vi "sub2.vi"(9 "Part References.Parse State Queue":refnum<vi>, 10 "regular expression":string, 11 "Array":T1(array[cluster])) -> (3 "Tunnel out":refnum<vi>)   [LabVIEW 2017, in "CSM-Helper.lvclass"]
doc: "### sub2.vi\n\n-- <b>Controls</b> --\n- <b>Part References.Parse State Queue</b>:\n- <b>regular expression</b>:\n- <b>Array</b>:\n\n-- <b>Indicators</b> --\n- <b>Tunnel out</b>:"
uses:
  CSM-Helper.lvclass
panel:
  # "Connector Pane"
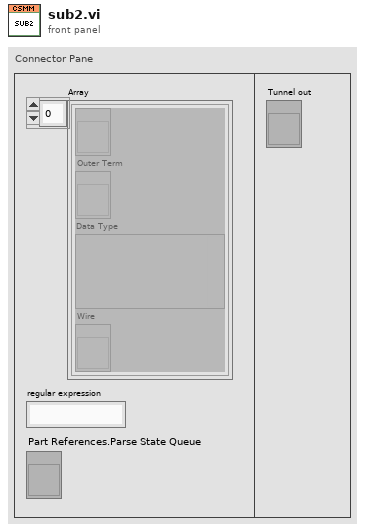
[diagram p1: front panel]
types:
  T1 = cluster{refnum<vi>, "Outer Term":refnum<vi>, "Data Type":variant, "Wire":refnum<vi>}[]
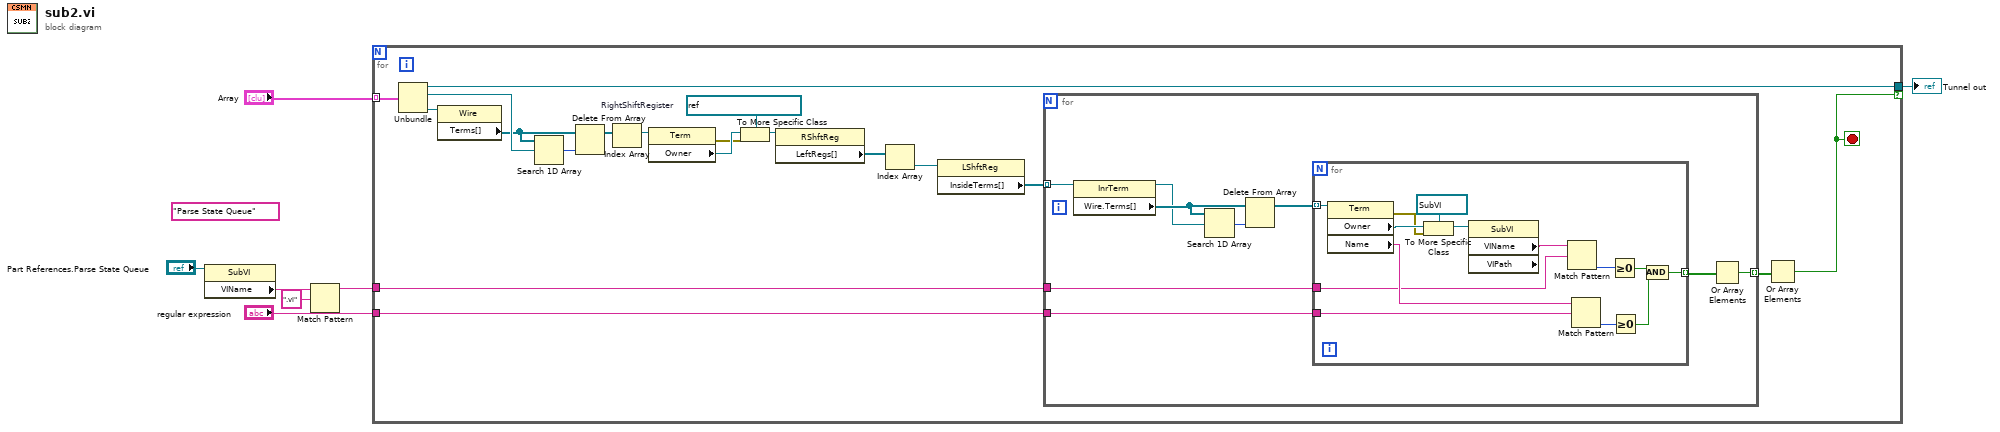
[diagram p0: block diagram]
diagram:
  (unwired) "Parse State Queue" ("regular expression")
  n1 = property class="SubVI"(reference="Part References.Parse State Queue") -> ("VIName"=w3:string)  [unwired: 1 in, 2 out]
  n2 = Match Pattern(string=w3, regular expression=".vi") -> (before substring=w2:string)  [unwired: 1 in, 3 out]
  n3 = for {
    tunnel: "Array" -> [w26] mode=indexing
    tunnel: [w25] -> w7 if=w16
    tunnel: "regular expression" -> [w15]
    tunnel: w2 -> [w8]
    stop <- w16 stop-if-true
    w22 = refnum<vi> refnum  # RightShiftRegister
    n4 = Unbundle(w26) -> (w25:refnum<vi>, "Outer Term"=w12:refnum<vi>, "Wire"=w24:refnum<vi>)  [unwired: 1 out]
    n5 = property class="Wire"(reference=w24) -> ("Terms[]"=w10:refnum<vi>[])  [unwired: 1 in, 2 out]
    n6 = Search 1D Array(1D array=w10, element=w12) -> (index of element=w11:i32)  [unwired: 1 in]
    n7 = Delete From Array(array=w10, index=w11) -> (array with subset deleted=w9:refnum<vi>[])  [unwired: 1 in, 1 out]
    n8 = Index Array(array=w9) -> (element=w23:refnum<vi>)  [unwired: 1 in]
    n9 = property class="Term"(reference=w23) -> (error out=w13:errorcluster, "Owner"=w14:refnum<vi>)  [unwired: 1 in, 1 out]
    n10 = To More Specific Class(target class=w22, reference=w14, error in=w13) -> (specific class reference=w21:refnum<vi>)  [unwired: 1 out]
    n11 = property class="RShftReg"(reference=w21) -> ("LeftRegs[]"=w20:refnum<vi>[])  [unwired: 1 in, 2 out]
    n12 = Index Array(array=w20) -> (element=w19:refnum<vi>)  [unwired: 1 in]
    n13 = property class="LShftReg"(reference=w19) -> ("InsideTerms[]"=w18:refnum<vi>[])  [unwired: 1 in, 2 out]
    n14 = for {
      tunnel: w18 -> [w35] mode=indexing
      tunnel: [w33] -> w17 mode=indexing
      tunnel: w15 -> [w32]
      tunnel: w8 -> [w27]
      n15 = property class="InrTerm"(reference=w35) -> (reference out=w28:refnum<vi>, "Wire.Terms[]"=w30:refnum<vi>[])  [unwired: 1 in, 1 out]
      n16 = Search 1D Array(1D array=w30, element=w28) -> (index of element=w31:i32)  [unwired: 1 in]
      n17 = Delete From Array(array=w30, index=w31) -> (array with subset deleted=w29:refnum<vi>[])  [unwired: 1 in, 1 out]
      n18 = for {
        tunnel: [w39] -> w34 mode=indexing
        tunnel: w29 -> [w38] mode=indexing
        tunnel: w32 -> [w37]
        tunnel: w27 -> [w36]
        n19 = property class="Term"(reference=w38) -> (error out=w47:errorcluster, "Owner"=w49:refnum<vi>, "Name"=w44:string)  [unwired: 1 in, 1 out]
        n20 = To More Specific Class(target class=refnum<vi> refnum ("Parse State Queue"), reference=w49, error in=w47) -> (specific class reference=w46:refnum<vi>)  [unwired: 1 out]
        n21 = property class="SubVI" props=["VIName", "VIPath"](reference=w46) -> ("VIName"=w45:string)  [unwired: 1 in, 3 out]
        n22 = Match Pattern(string=w45, regular expression=w36) -> (offset past match=w43:i32)  [unwired: 1 in, 3 out]
        n23 = Match Pattern(string=w44, regular expression=w37) -> (offset past match=w42:i32)  [unwired: 1 in, 3 out]
        n24 = Greater Or Equal To 0?(x=w43) -> (x >= 0?=w41:bool)
        n25 = Greater Or Equal To 0?(x=w42) -> (x >= 0?=w40:bool)
        n26 = And(x=w41, y=w40) -> (x .and. y?=w39:bool)
      }
      n27 = Or Array Elements(Boolean array=w34) -> (logical OR=w33:bool)
    }
    n28 = Or Array Elements(Boolean array=w17) -> (logical OR=w16:bool)
  }
  "Tunnel out" <- w7
